vi "LCD_WRITE_BUFFER.vi"(8 "error in (no error)":errorcluster, 11 "input_buffer":u8[](array[numeric])) -> (0 "error out":errorcluster)   [LabVIEW 2017]
uses:
  <vilib>/myRIO/Instrument Drivers/Onboard IO/I2C/typedefs/I2C User Configuration.ctl
  <vilib>/myRIO/Instrument Drivers/Onboard IO/I2C/typedefs/I2C Transfer Rate.ctl
  <vilib>/myRIO/Instrument Drivers/Onboard IO/I2C/typedefs/I2C Reference.ctl
  <vilib>/myRIO/Common/Instrument Driver Framework/Utilities/typedefs/myRIO Generic Hardware Reference.ctl
  <vilib>/myRIO/Common/Instrument Driver Framework/Utilities/typedefs/Hardware Version Enum.ctl
  <vilib>/myRIO/Common/Instrument Driver Framework/Utilities/typedefs/myRIO v1.0 Reference.ctl
  <vilib>/myRIO/Common/Instrument Driver Framework/Utilities/typedefs/Generic FPGA Reference.ctl
  <vilib>/myRIO/Common/Instrument Driver Framework/myRIO v1.0/I2C/typedefs/I2C Channels Enum.ctl
  <vilib>/myRIO/Instrument Drivers/Onboard IO/I2C/typedefs/I2C Configuration.ctl
  <vilib>/userdefined/High Color/nirio_resource_hc.ctl
  <vilib>/myRIO/Common/Instrument Driver Framework/Utilities/vis/Is FPGA Ref Available.vi
  <vilib>/myRIO/Common/Instrument Driver Framework/myRIO v1.0/I2C/vis/myRIO v1.1 Open I2C.vi
  <vilib>/myRIO/Instrument Drivers/Onboard IO/I2C/vis/Configure.vi
  <vilib>/myRIO/Instrument Drivers/Onboard IO/I2C/vis/Write.vi
  <vilib>/myRIO/Common/Instrument Driver Framework/Utilities/vis/Validate Channels.vi
  <vilib>/myRIO/Common/Instrument Driver Framework/myRIO v1.0/I2C/vis/myRIO v1.0 Reserve I2C.vi
  <vilib>/myRIO/Common/Instrument Driver Framework/myRIO v1.0/I2C/vis/myRIO v1.0 Build MUX Configuration I2C.vi
  <vilib>/myRIO/Common/Instrument Driver Framework/myRIO v1.0/Resource Manager/vis/myRIO v1.0 Reserve Channel List.vi
  <vilib>/myRIO/Common/Instrument Driver Framework/myRIO v1.0/Resource Manager/vis/myRIO v1.0 Create Configuration List.vi
  <vilib>/myRIO/Common/Instrument Driver Framework/myRIO v1.0/Resource Manager/vis/myRIO v1.0 Reserve Channel.vi
  <vilib>/myRIO/Common/Instrument Driver Framework/myRIO v1.0/Resource Manager/vis/myRIO v1.0 Unreserve Channel.vi
  <vilib>/myRIO/Common/Instrument Driver Framework/myRIO v1.0/Resource Manager/vis/myRIO v1.0 Build Mutex Name.vi
  <vilib>/Utility/VariantDataType/GetNumericInfo.vi
  <vilib>/Utility/error.llb/Error Cluster From Error Code.vi
  <vilib>/myRIO/Common/Instrument Driver Framework/myRIO v1.0/myRIO v1.1 Open.vi
  <vilib>/myRIO/Common/Instrument Driver Framework/Utilities/vis/IO Manager.vi
  <vilib>/myRIO/Common/Instrument Driver Framework/Utilities/vis/Configuration Manager.vi
  <vilib>/myRIO/Common/Instrument Driver Framework/myRIO v1.0/Resource Manager/vis/myRIO v1.0 Configure IO.vi
  <vilib>/myRIO/Common/Instrument Driver Framework/myRIO v1.0/myRIO v1.0 Close.vi
  <vilib>/myRIO/Common/Instrument Driver Framework/myRIO v1.0/I2C/vis/myRIO v1.0 Configure I2C.vi
  <vilib>/myRIO/Common/Instrument Driver Framework/myRIO v1.0/I2C/vis/myRIO v1.0 Write I2C.vi
  <vilib>/myRIO/Express VI/Onboard IO/I2C/I2C Express VI.xnode
  <vilib>/myRIO/Instrument Drivers/Onboard IO/I2C/vis/myRIO I2C Open.xnode
  <vilib>/myRIO/Instrument Drivers/Onboard IO/I2C/I2C.lvlib
panel:
  out "page_buffer":u8[](array[numeric])
  out "column":u8
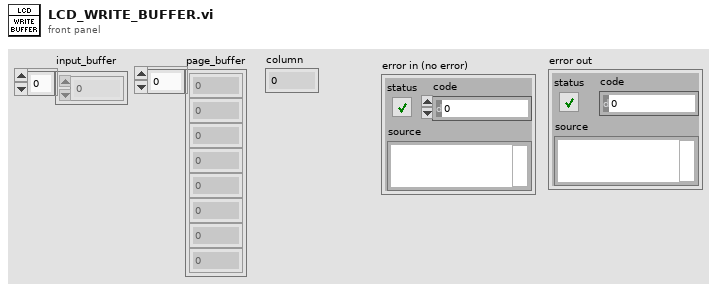
[diagram p1: front panel]
types:
  T1 = typedef "I2C.lvlib/I2C Reference.ctl" = cluster{"myRIO Reference":T2, "I2C Channels Enum":T6, "I2C Configuration":T7}
  T2 = typedef "myRIO Generic Hardware Reference.ctl" = cluster{"myRIO Model":T3, "myRIO Hardware Reference":T4}
  T3 = typedef "Hardware Version Enum.ctl" = enum16{"Unknown", "myRIO-1900", "myRIO-1950", "roboRIO", "NI ELVIS RIO CM"}
  T4 = typedef "myRIO v1.0 Reference.ctl" = cluster{"Generic FPGA Reference":T5, "Allow multiple opens":bool}
  T5 = typedef "Generic FPGA Reference.ctl" = refnum<k20>
  T6 = typedef "I2C Channels Enum.ctl" = enum16{"Not Connected", "A/I2C", "B/I2C", "I2C/I2C"}
  T7 = typedef "I2C.lvlib/I2C Configuration.ctl" = cluster{"I2C Transfer Rate":T8}
  T8 = typedef "I2C.lvlib/I2C Transfer Rate.ctl" = enum16{"Standard mode (100 kbps)", "Fast mode (400 kbps)"}
  T9 = typedef "I2C.lvlib/I2C User Configuration.ctl" = cluster{"I2C Transfer Rate":T8}
  T10 = typedef "nirio_resource_hc.ctl" = tag
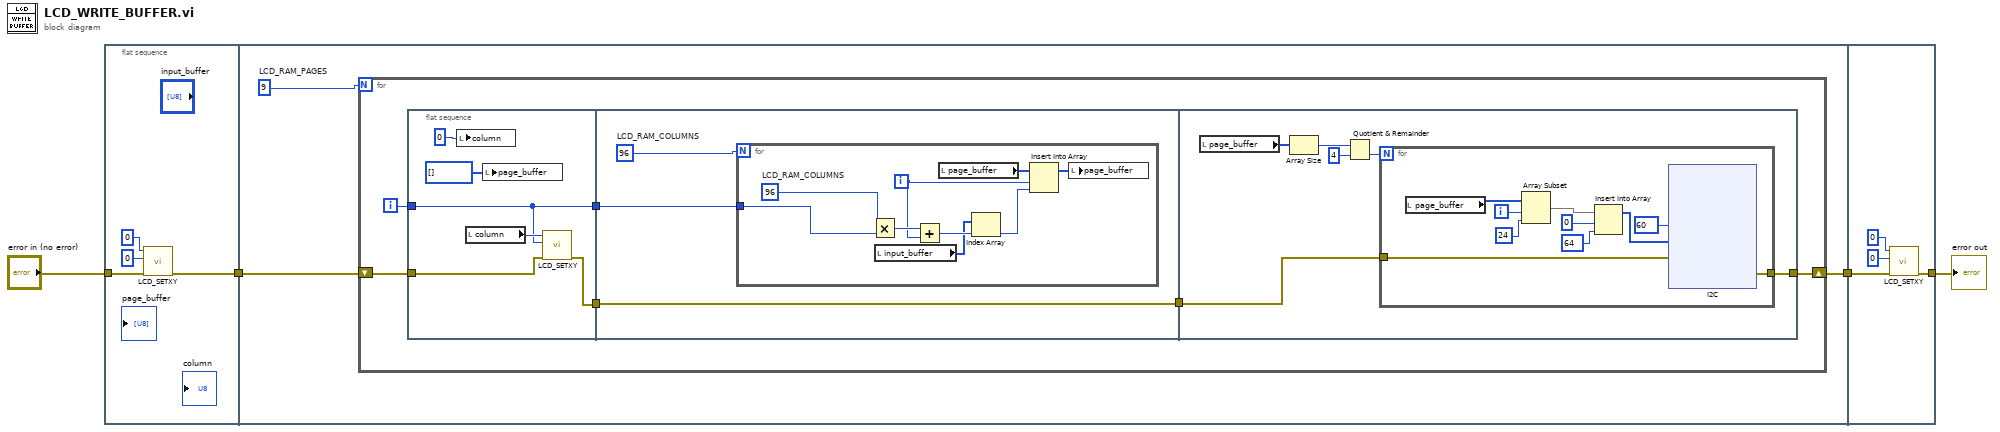
[diagram p0: block diagram]
diagram:
  n1 = flat-sequence {
    tunnel: [w6] -> w4
    tunnel: "error in (no error)" -> [w5]
    tunnel: w4 -> [w10]
    tunnel: [w9] -> w3
    tunnel: w3 -> [w91]
    tunnel: [w90] -> w2
    frame #0 {
      n2 = call "LCD_SETXY.vi"("error in (no error)"=w5, "y"=u8 0, "x"=u8 0) -> ("error out"=w6:errorcluster)  [unwired: 8 in]
    }
    frame #1 {
      w11 = u8 9  # LCD_RAM_PAGES
      n3 = for {
        N: w11 -> [_]
        shift-right: [w12] -> w9
        shift-left: w10 -> [w13]
        i -> [w17]
        n4 = flat-sequence {
          tunnel: w17 -> [w22]
          tunnel: [w22] -> w16
          tunnel: [w19] -> w14
          tunnel: w13 -> [w18]
          tunnel: w16 -> [w25]
          tunnel: [w24] -> w15
          tunnel: w14 -> [w24]
          tunnel: w15 -> [w37]
          tunnel: [w36] -> w12
          frame #0 {
            n5 = local write "column"(0 ("column")) -> ()
            n6 = local read "column"() -> (w23:u8)
            n7 = local write "page_buffer"(u8[] [] ("page_buffer")) -> ()
            n8 = call "LCD_SETXY.vi"("error in (no error)"=w18, "y"=w22, "x"=w23) -> ("error out"=w19:errorcluster)  [unwired: 8 in]
          }
          frame #1 {
            w26 = 96  # LCD_RAM_COLUMNS
            n9 = for {
              N: w26 -> [_]
              tunnel: w25 -> [w35]
              i -> [w29]
              w34 = 96  # LCD_RAM_COLUMNS
              n10 = Multiply(x=w34, y=w35) -> (x*y=w33:i32)
              n11 = local read "input_buffer"() -> (w31:u8[])
              n12 = Add(x=w33, y=w29) -> (x+y=w32:i32)
              n13 = local read "page_buffer"() -> (w28:u8[])
              n14 = Index Array "Index Array"(array=w31, index=w32) -> (element=w30:u8)
              n15 = Insert Into Array "Insert Into Array"(array=w28, index=w29, new element=w30) -> (w27:u8[])
              n16 = local write "page_buffer"(w27) -> ()
            }
          }
          frame #2 {
            n17 = local read "page_buffer"() -> (w39:u8[])
            n18 = Array Size(array=w39) -> (size(s)=w40:i32)
            n19 = Quotient & Remainder(x=w40, y=4) -> (floor(x/y)=w38:i32)  [unwired: 1 out]
            n20 = for {
              N: w38 -> [_]
              tunnel: w37 -> [w43]
              tunnel: [w42] -> w36
              i -> [w51]
              n21 = local read "page_buffer"() -> (w49:u8[])
              n22 = Array Subset "Array Subset"(array=w49, index=w51, length=24) -> (w48:u8[])
              n23 = Insert Into Array "Insert Into Array"(array=w48, index=0, new element=u8 64 ("new element/subarray")) -> (w45:u8[])
              n24 = xnode "I2C"("Slave Address (7-bit)"=u8 60, "Bytes to Write"=w45, "error in (no error)"=w43) -> ("error out"=w42:errorcluster)
            }
          }
        }
      }
    }
    frame #2 {
      n25 = call "LCD_SETXY.vi"("error in (no error)"=w91, "y"=u8 0, "x"=u8 0) -> ("error out"=w90:errorcluster)  [unwired: 8 in]
    }
  }
  "error out" <- w2
